vi "Show core.vi"(8 "error in (no error)":errorcluster, 11 "Subpanel in":refnum<class "Subpanel.lvclass">) -> (0 "error out":errorcluster)   [LabVIEW 2023, in "Panel Actor.lvlib" / "Panel.lvlib" / "Subpanel.lvclass"]
doc: "Inserts the VI in the sub panel.\n\n----\nPlease see the following web address for additional documentation and tutorial information:\nhttp://www.mooregoodideas.com/mgi-panel-manager/\n\nAuthor: Derek Trepanier\n\nCopyright (c) 2018, Moore Good Ideas, Inc.\n\nAll rights reserved.\n\nRedistribution and use in source and binary forms, with or without modification, are permitted provided that the following conditions are met:\n\n * Redistributions of source code must retain the above copyright notice, this list of conditions and the following disclaimer.\n * Redistributions in binary form must reproduce the above copyright notice, this list of conditions and the following disclaimer in the documentation and/or other materials provided with the distribution.\n * Neither the name of Moore Good Ideas, Inc. nor the names of its contributors may be used to endorse or promote products derived from this software without specific prior written permission.\n\nTHIS SOFTWARE IS PROVIDED BY THE COPYRIGHT HOLDERS AND CONTRIBUTORS \"AS IS\" AND ANY EXPRESS OR IMPLIED WARRANTIES, INCLUDING, BUT NOT LIMITED TO, THE IMPLIED WARRANTIES OF MERCHANTABILITY AND FITNESS FOR A PARTICULAR PURPOSE ARE DISCLAIMED. IN NO EVENT SHALL THE COPYRIGHT OWNER OR CONTRIBUTORS BE LIABLE FOR ANY DIRECT, INDIRECT, INCIDENTAL, SPECIAL, EXEMPLARY, OR CONSEQUENTIAL DAMAGES (INCLUDING, BUT NOT LIMITED TO, PROCUREMENT OF SUBSTITUTE GOODS OR SERVICES; LOSS OF USE, DATA, OR PROFITS; OR BUSINESS INTERRUPTION) HOWEVER CAUSED AND ON ANY THEORY OF LIABILITY, WHETHER IN CONTRACT, STRICT LIABILITY, OR TORT (INCLUDING NEGLIGENCE OR OTHERWISE) ARISING IN ANY WAY OUT OF THE USE OF THIS SOFTWARE, EVEN IF ADVISED OF THE POSSIBILITY OF SUCH DAMAGE."
uses:
  Subpanel.lvclass
  C:/Users/Public/Documents/Development/Engine/Panel Manager/Panel/Panel/Panel.lvclass
  Action.ctl
  Panel.lvclass/Panel.ctl
  Subpanel.lvclass/Subpanel.ctl
  Panel.lvclass
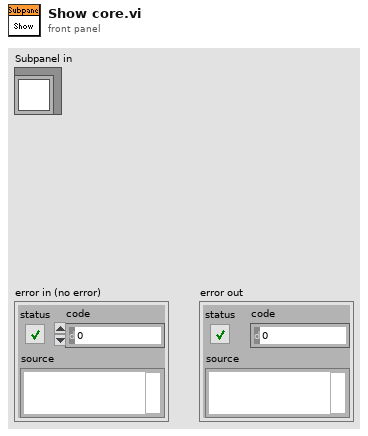
[diagram p1: front panel]
types:
  T1 = typedef "Panel Actor.lvlib/Panel.lvlib/Subpanel.lvclass/Action.ctl" = enum16{"Query", "Take", "Release"}
  T2 = typedef "Semaphore RefNum" = refnum<k1>
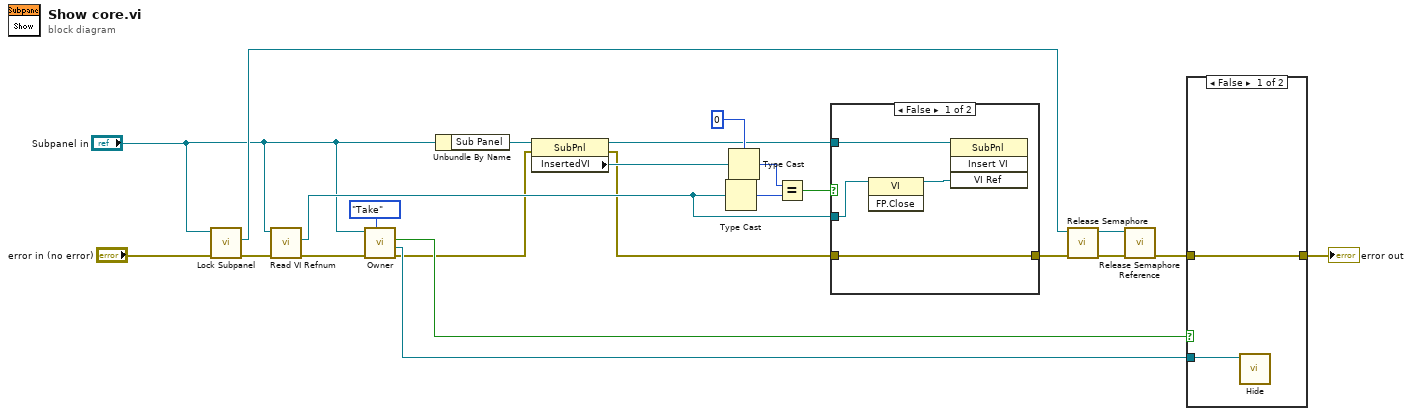
[diagram p0: block diagram]
diagram:
  w8 = u32 0
  n1 = call "Lock Subpanel.vi"("error in (no error)"="error in (no error)", "Subpanel in"="Subpanel in") -> ("error out"=w22:errorcluster, "semaphore"=w18:T2)  [unwired: 8 in]
  n2 = call "Read VI Refnum.vi"("error in (no error)"=w22, "Panel in"="Subpanel in") -> ("error out"=w21:errorcluster, "VI Refnum"=w20:refnum<vi>)  [unwired: 8 in]
  n3 = call "Owner.vi"("Action"=Action."Take", "error in (no error)"=w21, "Subpanel in"="Subpanel in") -> ("error out"=w6:errorcluster, "Old Owner"=w14:refnum<class "Panel.lvclass">, "I Was Owner?"=w15:bool)  [unwired: 6 in]
  n4 = Unbundle By Name("Subpanel in") -> ("Sub Panel"=w13:refnum<vi>)
  n5 = property class="SubPnl"(reference=w13, error in=w6) -> (reference out=w7:refnum<vi>, error out=w4:errorcluster, "InsertedVI"=w12:refnum<vi>)
  n6 = Type Cast(type=w8, x=w20) -> (*(type *) &x=w10:u32)
  n7 = Type Cast(type=w8, x=w12) -> (*(type *) &x=w11:u32)
  n8 = Equal?(x=w11, y=w10) -> (x = y?=w9:bool)
  n9 = case shown="False" w9 {
    tunnel: w7 -> [w27 _]
    tunnel: w20 -> [w26 _]
    tunnel: [w24 w28] -> w5
    tunnel: w4 -> [w24 w28]
    frame False {
      n10 = invoke class="VI" method="FP.Close"(reference=w26) -> (reference out=w25:refnum<vi>)  [unwired: 2 in, 2 out]
      n11 = invoke class="SubPnl" method="Insert VI"(reference=w27, "VI Ref"=w25) -> ()  [unwired: 2 in, 4 out]
    }
    frame True {
      # "Already properly inserted"
    }
  }
  n12 = call <vilib>:"Release Semaphore.vi"("error in (no error)"=w5, "semaphore"=w18) -> ("error out"=w3:errorcluster, "semaphore out"=w2:T2)  [unwired: 4 in]
  n13 = call <vilib>:"Release Semaphore Reference.vi"("error in (no error)"=w3, "semaphore"=w2) -> ("error out"=w1:errorcluster)  [unwired: 8 in, 1 out]
  n14 = case shown="False" w15 {
    tunnel: w1 -> [w29 w31]
    tunnel: [w29 w31] -> w16
    tunnel: w14 -> [w30 _]
    frame False {
      n15 = call "Hide.vi"("Panel In"=w30) -> ()  [unwired: 10 in, 1 out]
    }
    frame True {
    }
  }
  "error out" <- w16
